vi "AlarmGetList.vi"() -> (0 "error out":errorcluster, 2 "alarms":string[](array[string]))   [LabVIEW 2015, in "ni-veristand-steps-runtime-lib.lvlib"]
uses:
  ni-veristand-steps-runtime-lib.lvlib
  <vilib>/NI Veristand/Execution/AlarmManager/NI_VS AlarmManager ExecutionAPI.lvlib
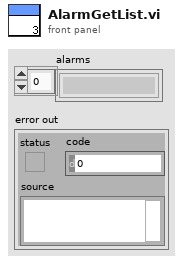
[diagram p1: front panel]
types:
  T1 = typedef "ni-veristand-steps-runtime-lib.lvlib/VeriStand dotNet References.ctl" = cluster{"Project Ref":refnum<k24>, "Workspace Manager Ref":refnum<k24>, "Model Manager Ref":refnum<k24>, "Channel Fault Manager Ref":refnum<k24>, "Alarm Manager Ref":refnum<k24>}
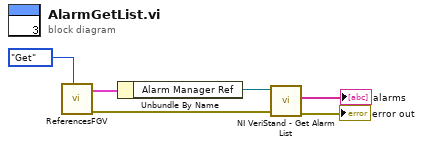
[diagram p0: block diagram]
diagram:
  n1 = call "ReferencesFGV.vi"("Get/Set"=enum16{"Get", "Set"}."Get") -> ("error out"=w3:errorcluster, "VeriStand dotNET Refs out"=w5:T1)  [unwired: 9 in]
  n2 = Unbundle By Name(w5) -> ("Alarm Manager Ref"=w4:refnum<k24>)
  n3 = call <vilib>:"NI VeriStand - Get Alarm List.vi"("error in (no error)"=w3, "AlarmManager in"=w4) -> ("error out"=→"error out":errorcluster, "alarms"=→"alarms":string[])  [unwired: 7 in, 1 out]
